vi "globale Variable 1.vi"() -> ()   [LabVIEW 2010]
panel:
  in  "not-aus?":bool
  in  "ende?":bool
  in  "error in (no error)":errorcluster caption="Fehler (Eingang, kein Fehler)"
  in  "licht an?":bool
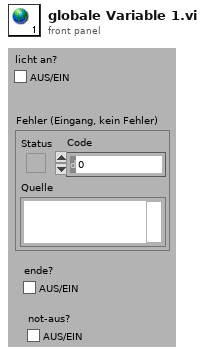
[diagram p1: front panel]
diagram:
